vi "Begin.vi"(8 "error in":errorcluster) -> (0 "error out":errorcluster)   [LabVIEW 2017]
doc: "Called before other user functions, this VI is expected to open initial I/O refnums, load in file data, and do all program initialization. Notice that the <B>error out</B> terminal is simply used for data flow. Wiring it to other structures or subVIs ensures that this VI runs first."
uses:
  <vilib>/Rock Robotics/WPI/DriverStation/WPI_DriverStationRobotMode2.ctl
  <vilib>/Rock Robotics/WPI/Joystick/WPI_JoystickDeviceEnum.ctl
  <vilib>/Rock Robotics/WPI/Solenoid/WPI_SolenoidChannel.ctl
  <vilib>/Rock Robotics/WPI/Solenoid/WPI_SolenoidValue.ctl
  <vilib>/Rock Robotics/SystemInterfaces/spilib/spi_bus.ctl
  Main/Robot Global Data.vi
  <vilib>/Rock Robotics/Network Tables/NT Write String Array.vi
  <vilib>/Rock Robotics/WPI/Solenoid/WPI_SolenoidOpenDouble.vi
  <vilib>/Rock Robotics/WPI/Solenoid/WPI_SolenoidOpenSingle.vi
  <vilib>/Rock Robotics/WPI/Solenoid/WPI_SolenoidSetEnum.vi
  <vilib>/Rock Robotics/WPI/Utilities/WPI_GetSetVariantRefNum.vi
  <vilib>/Rock Robotics/WPI/Gyro/WPI_GyroXRS450_SPI_Open.vi
  <vilib>/Rock Robotics/WPI/ThirdParty/Sensors/navX/_TypeDefs/FRIC_navX_DeviceNumbersTypeDef.ctl
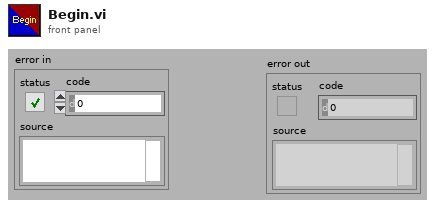
[diagram p1: front panel]
types:
  T1 = typedef "spi_bus.ctl" = enum16{"SPI On-Board, CS0", "SPI On-Board, CS1", "SPI On-Board, CS2", "SPI On-Board, CS3", "SPI MXP", "Invalid"}
  T2 = typedef "WPI_SolenoidValue.ctl" = enum16{"Off", "On", "Forward", "Reverse"}
  T3 = typedef "WPI_SolenoidChannel.ctl" = enum8{"Solenoid 0", "Solenoid 1", "Solenoid 2", "Solenoid 3", "Solenoid 4", "Solenoid 5", "Solenoid 6", "Solenoid 7", "Invalid"}
  T4 = typedef "WPI_JoystickDeviceEnum.ctl" = enum16{"USB 0", "USB 1", "USB 2", "USB 3", "USB 4", "USB 5"}
  T5 = typedef "WPI_DriverStationRobotMode2.ctl" = enum16{"Autonomous Disabled", "Autonomous Enabled", "Teleop Disabled", "Teleop Enabled", "Disconnected", "Finish", "Test Disabled", "Test Enabled", "Emergency Stopped"}
  T6 = typedef "WPI_JoystickDevRef.ctl" = cluster{"Device":T4}
  T7 = typedef "WPI_CompressorDevRef.ctl" = cluster{"DevStatus":errorcluster, "Pneumatics Control Module":u8}
  T8 = typedef "WPI_GyroDevRef.ctl" = cluster{"DevStatus":errorcluster, "Analog Channel":T9, "Gain (VoltsPerDegree/Second)":dbl, "Gyro Type":enum16{"Analog", "XRS450"}, "Handle":i32, "SPI Bus":T1, "Device Found":bool, "Sample Rate":dbl, "Calibrate On Open":bool, "Offset":dbl}
  T9 = typedef "FPGA_AIChannel.ctl" = enum8{"AI 0", "AI 1", "AI 2", "AI 3", "AI MXP 0", "AI MXP 1", "AI MXP 2", "AI MXP 3", "Invalid"}
  T10 = typedef "WPI_SolenoidDevRef.ctl" = cluster{"DevStatus":errorcluster, "Pneumatics Control Module":u8, "Forward Solenoid Channel":T3, "Reverse Solenoid Channel":T3}
  T11 = typedef "FRIC_navX_DeviceNumbersTypeDef.ctl" = enum16{"Dev0", "Dev1", "Dev2", "Dev3"}
  T12 = typedef "WPI_MotorControlDeviceRef.ctl" = cluster{"DeviceStatus":errorcluster, "Type":T13, "PWM":cluster{"PWM Channel":T14, "DeadBand":T15}, "CAN":cluster{"Device Number":u8, "SetOutput VI Ref":variant, "GetOutput VI Ref":variant, "Enable VI Ref":variant, "Disable VI Ref":variant, "Data":variant}, "Invert":bool, "DIO PWM":cluster{"PWM \"Enable\" Channel":T14, "DIOChannel":T16, "PWM Rate":dbl}}
  T13 = typedef "WPI_MotorControlType.ctl" = enum16{"PWM", "CAN", "DIO PWM"}
  T14 = typedef "FPGA_DIOPWMChannel.ctl" = enum8{"PWM 0", "PWM 1", "PWM 2", "PWM 3", "PWM 4", "PWM 5", "PWM 6", "PWM 7", "PWM 8", "PWM 9", "PWM MXP 0", "PWM MXP 1", "PWM MXP 2", "PWM MXP 3", "PWM MXP 4", "PWM MXP 5", "PWM MXP 6", "PWM MXP 7", "PWM MXP 8", "PWM MXP 9", "Invalid"}
  T15 = typedef "WPI_PWMDeadband.ctl" = cluster{"Name":string, "maxPositivePwm":i32, "minPositivePwm":i32, "centerPwm":i32, "maxNegativePwm":i32, "minNegativePwm":i32, "angularRange":u16}
  T16 = typedef "FPGA_DIOChannel.ctl" = enum8{"DIO 0", "DIO 1", "DIO 2", "DIO 3", "DIO 4", "DIO 5", "DIO 6", "DIO 7", "DIO 8", "DIO 9", "DIO MXP 0", "DIO MXP 1", "DIO MXP 2", "DIO MXP 3", "DIO MXP 4", "DIO MXP 5", "DIO MXP 6", "DIO MXP 7", "DIO MXP 8", "DIO MXP 9", "DIO MXP 10", "DIO MXP 11", "DIO MXP 12", "DIO MXP 13", "DIO MXP 14", "DIO MXP 15", "SPI Port CS1", "SPI Port CS2", "SPI Port CS3", "SPI Port MISO", "SPI Port MOSI", "Invalid"}
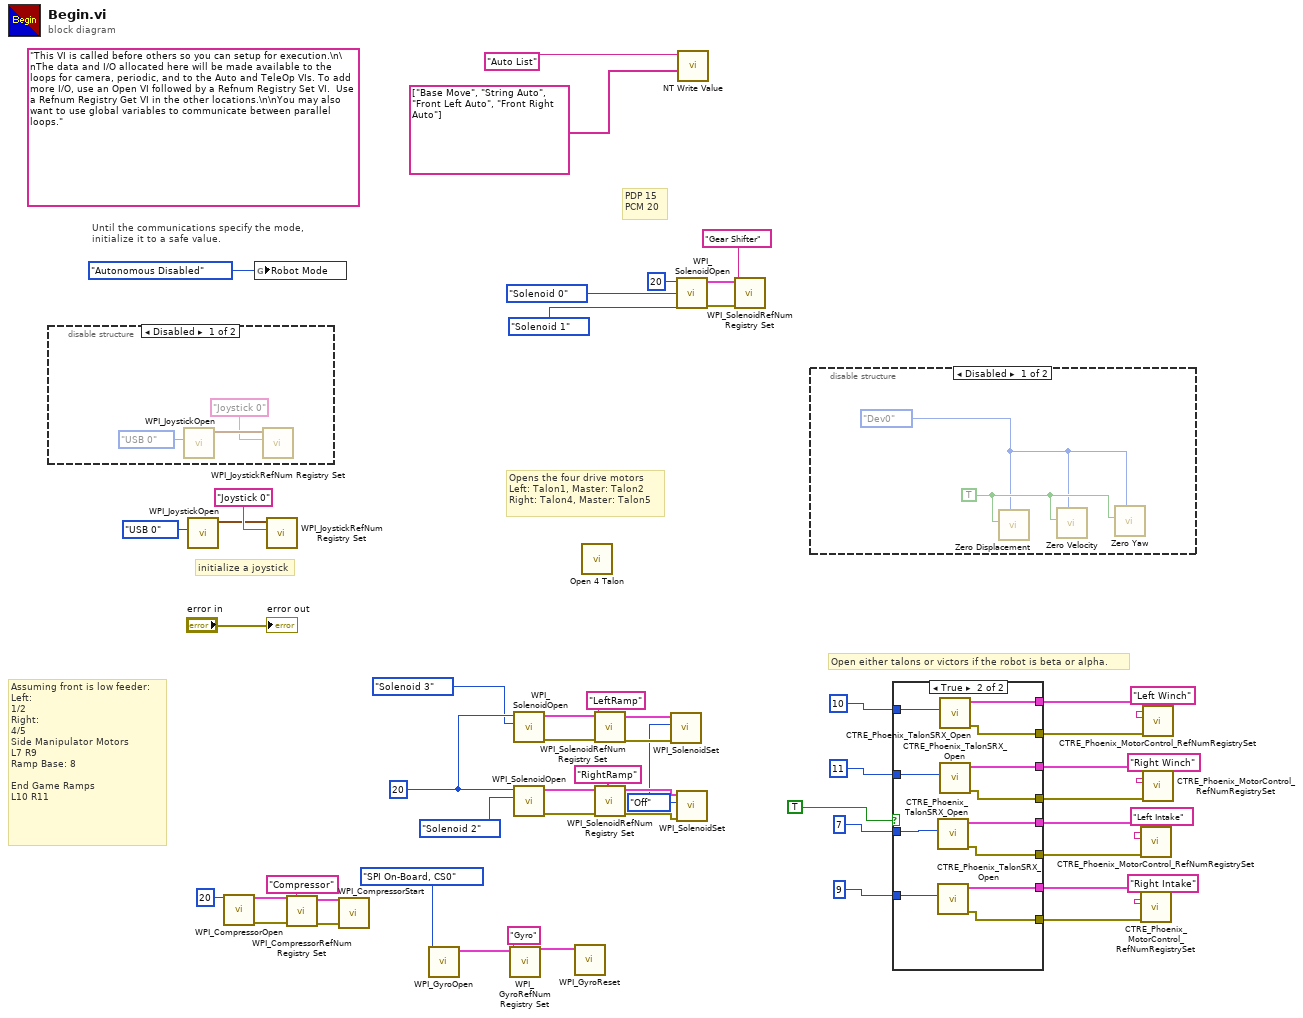
[diagram p0: block diagram]
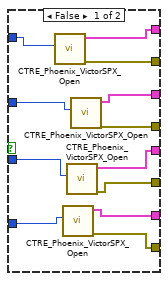
[diagram p4: hidden frame]
diagram:
  w28 = WPI_SolenoidValue."Off" ("Value")
  w35 = u8 20 ("Pneumatics Control Module (0)")
  (unwired) "This VI is called before others so you can setup for execution.\n\nThe data and I/O allocated here will be made available to the loops for camera, periodic, and to the Auto and TeleOp VIs. To add more I/O, use an Open VI followed by a Refnum Registry Set VI.  Use a Refnum Registry Get VI in the other locations.\n\nYou may also want to use global variables to communicate between parallel loops."
  # "Open either talons or victors if the robot is beta or alpha."
  # "Opens the four drive motors\nLeft: Talon1, Master: Talon2\nRight: Talon4, Master: Talon5"
  # "Assuming front is low feeder:\nLeft:\n1/2\nRight:\n4/5\nSide Manipulator Motors\nL7 R9\nRamp Base: 8\n\nEnd Game Ramps\nL10 R11"
  # "PDP 15\nPCM 20"
  # "initialize a joystick"
  # "Until the communications specify the mode,\ninitialize it to a safe value."
  n1 = disable-structure shown="Disabled" {
    frame Disabled {
      n2 = call <vilib>:"WPI_JoystickOpen.vi"("JoystickDevice"=WPI_JoystickDeviceEnum."USB 0") -> ("JoystickDevRef"=w56:T6)  [unwired: 10 in]
      n3 = call <vilib>:"WPI_JoystickRefNum Registry Set.vi"("refnum name"="Joystick 0", "JoystickDevRef"=w56) -> ()  [unwired: 8 in, 2 out]
    }
    frame Enabled {
    }
  }
  n4 = call <vilib>:"WPI_JoystickOpen.vi"("JoystickDevice"=WPI_JoystickDeviceEnum."USB 0") -> ("JoystickDevRef"=w52:T6)  [unwired: 10 in]
  n5 = call <vilib>:"WPI_CompressorOpen.vi"("Pneumatics Control Module (0)"=u8 20) -> ("CompressorDevRef"=w8:T7, "error out"=w7:errorcluster)  [unwired: 13 in]
  n6 = global write "Robot Global Data.vi" "Robot Mode"(WPI_DriverStationRobotMode2."Autonomous Disabled" ("Robot Mode")) -> ()
  n7 = call <vilib>:"WPI_JoystickRefNum Registry Set.vi"("refnum name"="Joystick 0", "JoystickDevRef"=w52) -> ()  [unwired: 8 in, 2 out]
  n8 = call <vilib>:"WPI_CompressorRefNum Registry Set.vi"("error in (no error)"=w7, "refnum name"="Compressor", "CompressorDevRef"=w8) -> ("error out"=w10:errorcluster, "CompressorDevRef"=w9:T7)  [unwired: 7 in]
  n9 = call <vilib>:"WPI_CompressorStart.vi"("error in (no error)"=w10, "CompressorDevRef"=w9) -> ()  [unwired: 8 in, 2 out]
  n10 = call-poly <vilib>:"WPI_GyroOpen.vi"("SPI Bus"=spi_bus."SPI On-Board, CS0") -> ("GyroDevRef"=w4:T8)  [unwired: 8 in, 2 out]
  n11 = call <vilib>:"WPI_GyroRefNum Registry Set.vi"("refnum name"="Gyro", "GyroDevRef"=w4) -> ("GyroDevRef"=w3:T8)  [unwired: 8 in, 1 out]
  n12 = call-poly <vilib>:"WPI_SolenoidOpen.vi"("Solenoid Channel"=WPI_SolenoidChannel."Solenoid 3", "Pneumatics Control Module (0)"=w35) -> ("error out"=w40:errorcluster, "SolenoidDevRef"=w41:T10)  [unwired: 8 in]
  n13 = call-poly <vilib>:"WPI_SolenoidOpen.vi"("Solenoid Channel"=WPI_SolenoidChannel."Solenoid 2", "Pneumatics Control Module (0)"=w35) -> ("error out"=w38:errorcluster, "SolenoidDevRef"=w39:T10)  [unwired: 8 in]
  n14 = call <vilib>:"WPI_GyroReset.vi"("GyroDevRef"=w3) -> ()  [unwired: 9 in, 2 out]
  n15 = call "Open 4 Talon.vi"() -> ()  [unwired: 12 in]
  n16 = call <vilib>:"WPI_SolenoidRefNum Registry Set.vi"("error in (no error)"=w40, "refnum name"="LeftRamp", "SolenoidDevRef"=w41) -> ("error out"=w31:errorcluster, "SolenoidDevRef"=w32:T10)  [unwired: 7 in]
  n17 = call <vilib>:"WPI_SolenoidRefNum Registry Set.vi"("error in (no error)"=w38, "refnum name"="RightRamp", "SolenoidDevRef"=w39) -> ("error out"=w29:errorcluster, "SolenoidDevRef"=w30:T10)  [unwired: 7 in]
  n18 = call-poly <vilib>:"WPI_SolenoidSet.vi"("error in (no error)"=w31, "Value"=w28, "SolenoidDevRef"=w32) -> ()  [unwired: 7 in, 2 out]
  n19 = call-poly <vilib>:"WPI_SolenoidOpen.vi"("Reverse Solenoid Channel"=WPI_SolenoidChannel."Solenoid 1", "Forward Solenoid Channel"=WPI_SolenoidChannel."Solenoid 0" ("Solenoid Channel"), "Pneumatics Control Module (0)"=u8 20) -> ("error out"=w45:errorcluster, "SolenoidDevRef"=w44:T10)  [unwired: 7 in]
  n20 = call-poly <vilib>:"WPI_SolenoidSet.vi"("error in (no error)"=w29, "Value"=w28, "SolenoidDevRef"=w30) -> ()  [unwired: 7 in, 2 out]
  n21 = call-poly <vilib>:"NT Write Value.vi"("String Array"=string[] ["Base Move", "String Auto", "Front Left Auto", "Front Right Auto"], "Name"="Auto List") -> ()  [unwired: 9 in, 1 out]
  n22 = call <vilib>:"WPI_SolenoidRefNum Registry Set.vi"("error in (no error)"=w45, "refnum name"="Gear Shifter", "SolenoidDevRef"=w44) -> ()  [unwired: 7 in, 2 out]
  n23 = disable-structure shown="Disabled" {
    frame Disabled {
      w58 = FRIC_navX_DeviceNumbersTypeDef."Dev0" ("Device Number")
      w59 = TRUE ("Zero")
      n24 = call <vilib>:"Zero Displacement.vi"("Device Number"=w58, "Zero"=w59) -> ()  [unwired: 10 in]
      n25 = call <vilib>:"Zero Velocity.vi"("Device Number"=w58, "Zero"=w59) -> ()  [unwired: 10 in]
      n26 = call <vilib>:"Zero Yaw.vi"("Device Number"=w58, "Zero"=w59) -> ()  [unwired: 10 in]
    }
    frame Enabled {
    }
  }
  n27 = case shown="True" TRUE ("Beta?") {
    tunnel: [w63 w83] -> w27
    tunnel: [w64 w82] -> w25
    tunnel: [w62 w81] -> w24
    tunnel: [w61 w80] -> w22
    tunnel: [w69 w79] -> w21
    tunnel: [w70 w78] -> w19
    tunnel: [w68 w77] -> w18
    tunnel: [w67 w76] -> w16
    tunnel: u8 11 ("Device Number") -> [w65 w75]
    tunnel: u8 10 ("Device Number") -> [w60 w74]
    tunnel: u8 9 ("Device Number") -> [w71 w73]
    tunnel: u8 7 ("Device Number") -> [w66 w72]
    frame False {
      n28 = call <vilib>:"CTRE_Phoenix_VictorSPX_Open.vi"("Device Number"=w60) -> ("error out"=w62:errorcluster, "CAN Talon SRX Ref"=w61:T12)  [unwired: 9 in]
      n29 = call <vilib>:"CTRE_Phoenix_VictorSPX_Open.vi"("Device Number"=w71) -> ("error out"=w69:errorcluster, "CAN Talon SRX Ref"=w70:T12)  [unwired: 9 in]
      n30 = call <vilib>:"CTRE_Phoenix_VictorSPX_Open.vi"("Device Number"=w66) -> ("error out"=w68:errorcluster, "CAN Talon SRX Ref"=w67:T12)  [unwired: 9 in]
      n31 = call <vilib>:"CTRE_Phoenix_VictorSPX_Open.vi"("Device Number"=w65) -> ("error out"=w63:errorcluster, "CAN Talon SRX Ref"=w64:T12)  [unwired: 9 in]
    }
    frame True {
      n32 = call <vilib>:"CTRE_Phoenix_TalonSRX_Open.vi"("Device Number"=w72) -> ("error out"=w77:errorcluster, "CAN Talon SRX Ref"=w76:T12)  [unwired: 9 in]
      n33 = call <vilib>:"CTRE_Phoenix_TalonSRX_Open.vi"("Device Number"=w73) -> ("error out"=w79:errorcluster, "CAN Talon SRX Ref"=w78:T12)  [unwired: 9 in]
      n34 = call <vilib>:"CTRE_Phoenix_TalonSRX_Open.vi"("Device Number"=w74) -> ("error out"=w81:errorcluster, "CAN Talon SRX Ref"=w80:T12)  [unwired: 9 in]
      n35 = call <vilib>:"CTRE_Phoenix_TalonSRX_Open.vi"("Device Number"=w75) -> ("error out"=w83:errorcluster, "CAN Talon SRX Ref"=w82:T12)  [unwired: 9 in]
    }
  }
  n36 = call <vilib>:"CTRE_Phoenix_MotorControl_RefNumRegistrySet.vi"("error in (no error)"=w18, "refnum name"="Left Intake", "PhoenixMotorControlDevRef"=w16) -> ()  [unwired: 7 in, 2 out]
  n37 = call <vilib>:"CTRE_Phoenix_MotorControl_RefNumRegistrySet.vi"("error in (no error)"=w21, "refnum name"="Right Intake", "PhoenixMotorControlDevRef"=w19) -> ()  [unwired: 7 in, 2 out]
  n38 = call <vilib>:"CTRE_Phoenix_MotorControl_RefNumRegistrySet.vi"("error in (no error)"=w24, "refnum name"="Left Winch", "PhoenixMotorControlDevRef"=w22) -> ()  [unwired: 7 in, 2 out]
  n39 = call <vilib>:"CTRE_Phoenix_MotorControl_RefNumRegistrySet.vi"("error in (no error)"=w27, "refnum name"="Right Winch", "PhoenixMotorControlDevRef"=w25) -> ()  [unwired: 7 in, 2 out]
  "error out" <- "error in"
